vi "Add Spatial Temporal Folder Path.vi"(8 "Shot Number":dbl, 9 "cameraselect":enum16{"temporal CAM", "spatial CAM"}(ring), 11 "Input Path":path) -> (3 "Output Path":path)   [LabVIEW 2020]
panel:
  out "concatenated string":string
  out "ShotNumber":string
  out "DeviceName":string
  out "match + rest of string":string
  out "Scan Number":string
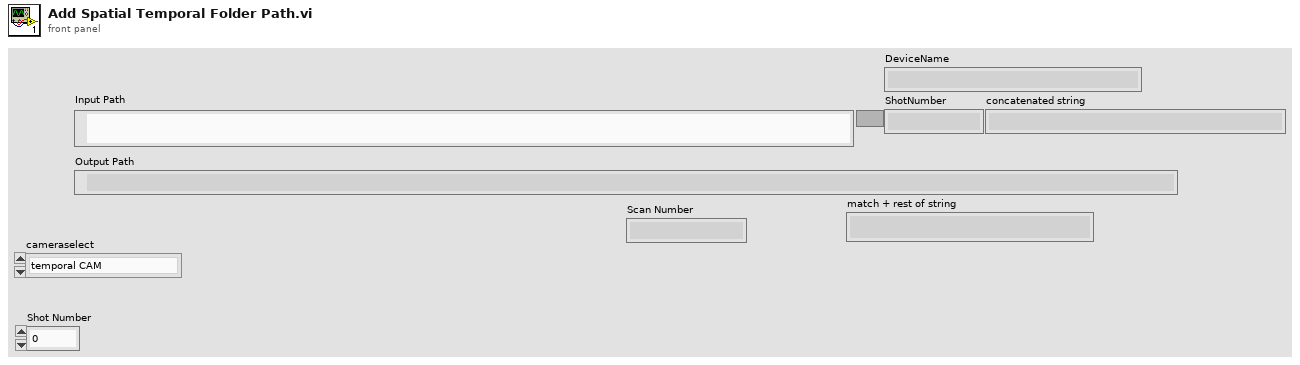
[diagram p1: front panel]
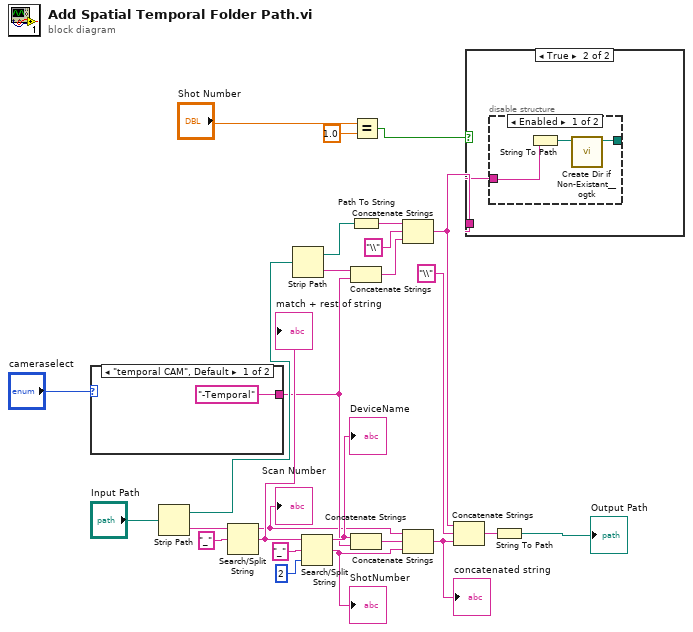
[diagram p0: block diagram]
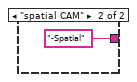
[diagram p4: hidden frame]
diagram:
  n1 = case shown="\"temporal CAM\", Default" "cameraselect" {
    tunnel: ["-Temporal" ("string") "-Spatial" ("string")] -> w8
    frame "temporal CAM", Default {
    }
    frame "spatial CAM" {
    }
  }
  n2 = Strip Path(path="Input Path") -> (stripped path=w24:path, name=w14:string)
  n3 = Search/Split String(string=w14, search string/char (-)="_") -> (substring before match=w7:string, match + rest of string=w11:string)  [unwired: 1 in, 1 out]
  "Scan Number" <- w7
  "match + rest of string" <- w11
  n4 = Strip Path(path=w24) -> (stripped path=w15:path, name=w25:string)
  n5 = Search/Split String(string=w11, search string/char (-)="_", offset (0)=2) -> (substring before match=w9:string, match + rest of string=w5:string)  [unwired: 1 out]
  "DeviceName" <- w9
  "ShotNumber" <- w5
  n6 = Path To String(path=w15) -> (string=w23:string)
  n7 = Concatenate Strings(w25, w8) -> (w21:string)
  n8 = Concatenate Strings(w9, w8) -> (w6:string)
  n9 = Equal?(x="Shot Number", y=1.0) -> (x = y?=w1:bool)
  n10 = Concatenate Strings(w23, "\\" ("string"), w21) -> (w19:string)
  n11 = Concatenate Strings(w7, w6, w5) -> (w4:string)
  "concatenated string" <- w4
  n12 = Concatenate Strings(w19, "\\" ("string"), w4) -> (w17:string)
  n13 = case shown="True" w1 {
    tunnel: w19 -> [_ w29]
    frame False {
    }
    frame True {
      n14 = disable-structure shown="Enabled" {
        disable-tunnel: w29 -> [w32 _]
        disable-tunnel: [w30 _] -> _
        frame Enabled {
          n15 = String To Path(string=w32) -> (path=w31:path)
          n16 = call <userlib>:"Create Dir if Non-Existant__ogtk.vi"("Directory Path"=w31) -> ("dup Directory Path"=w30:path)  [unwired: 8 in, 2 out]
        }
        frame Disabled {
        }
      }
    }
  }
  n17 = String To Path(string=w17) -> (path=→"Output Path":path)
